vi "Global_ACT_Data Out.vi"() -> ()   [LabVIEW 2023, in "Thor-SwerveDrive_ACT.lvlib"]
uses:
  Thor-SwerveDrive_ACT.lvlib
  Shared Code/TypeDefs/Cluster_FWD  REV Values.ctl
  Shared Code/TypeDefs/Cluster_High-Low.ctl
  Shared Code/TypeDefs/Cluster_PID Gains.ctl
  Shared Code/TypeDefs/Cluster_PID Config.ctl
  Shared Code/TypeDefs/Cluster_Config_Balance Data.ctl
panel:
  in  "ACT_Swerve_Position ft":dbl
  in  "ACT_SwerveDrive_Balance Config":T1={"BalancePID Ver"=0, "PID"={"Gains"={"P"=4.0, "I"=0.0, "D"=50.0, "F"=0.0}, "Error Allowed"={"High"=0.01, "Low"=-0.01}, "I Zone"={"High"=10.0, "Low"=-10.0}, "Max Out"={"FWD"=0.44, "REV"=-0.44}, "Max I Accu"={"High"=100000.0, "Low"=-100000.0}, "CL Ramp Rate (S)"=0.01}} {"PID"."Max I Accu"."Low" format="%#.8f"; "PID"."Max I Accu"."High" format="%#.8f"; "PID"."Gains"."F" format="%#.8f"; "PID"."Gains"."D" format="%#.8f"; "PID"."Gains"."I" format="%#.8f"; "PID"."Gains"."P" format="%#.8f"; "PID"."Error Allowed"."Low" format="%#.8f"; "PID"."Error Allowed"."High" format="%#.8f"; "PID"."I Zone"."Low" format="%#.8f"; "PID"."I Zone"."High" format="%#.8f"; "PID"."Max Out"."REV" format="%.2f"; "PID"."Max Out"."FWD" format="%.2f"}
  out "ACT_SwerveDrive_Balanced":bool
  in  "ACT_Drive_Distances_(ft)":dbl[](array[numeric])
  out "ACT_SwerveDrive_At Angle":bool
  out "ACT_SwerveDrive_At Position":bool
  in  "ACT_Swerve_CycleTime(S)":dbl
  in  "ACT_SwerveDrive_Directions":dbl[](array[numeric])
  # "The Names of the Data items in the Global Variable MUST describe who the Single Writer is\nFor Actuator Globals the the naming convention is\n   \nACT_Lib Name_Data Name\n\nExamples:\nACT_Drive_X axis\nACT_Hopper_AgitatorSpeed"
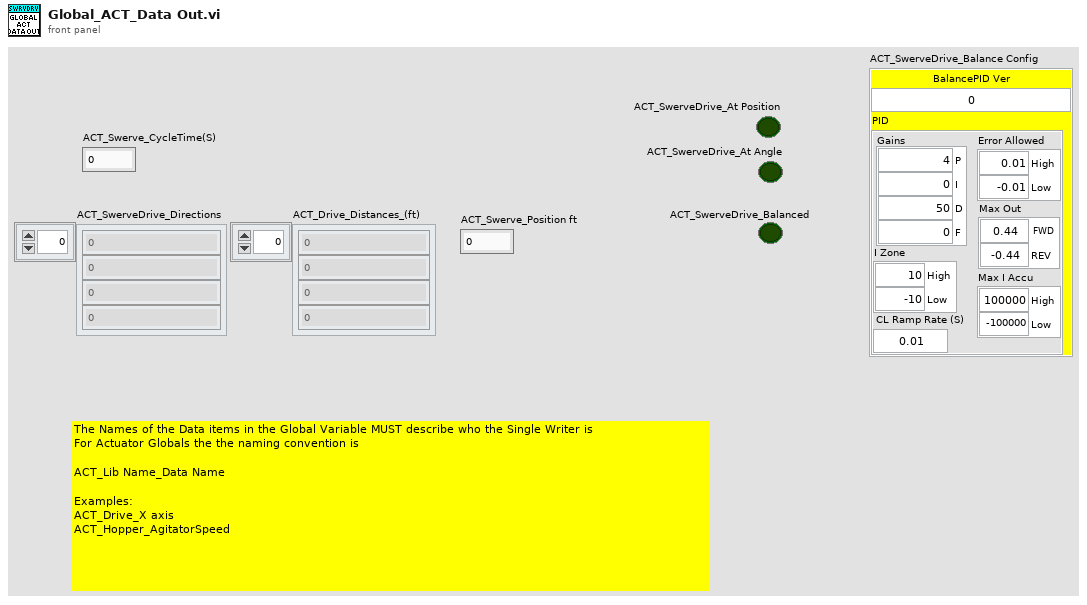
[diagram p1: front panel]
types:
  T1 = typedef "Cluster_Config_Balance Data.ctl" = cluster{"BalancePID Ver":u64, "PID":T2}
  T2 = typedef "Cluster_PID Config.ctl" = cluster{"Gains":T3, "Error Allowed":T4, "I Zone":T4, "Max Out":T5, "Max I Accu":T4, "CL Ramp Rate (S)":dbl}
  T3 = typedef "Cluster_PID Gains.ctl" = cluster{"P":dbl, "I":dbl, "D":dbl, "F":dbl}
  T4 = typedef "Cluster_High-Low.ctl" = cluster{"High":dbl, "Low":dbl}
  T5 = typedef "Cluster_FWD  REV Values.ctl" = cluster{"FWD":dbl, "REV":dbl}
diagram:
